vi "arm control.vi"(1 "State":T1, 2 "Z Axis (Tuning)":dbl) -> (0 "setpoint":dbl format="%.2f")   [LabVIEW 2013]
uses:
  typedefs/subStates.ctl
  typedefs/fg_typedef.ctl
panel:
  in  "lower limit":dbl=-0.015 format="%#_13g"
  in  "upper limit":dbl=0.015 format="%#_13g"
  in  "2nd Up setpoint":dbl format="%#_13g"
  in  "1st Up setpoint":dbl format="%#_13g"
  # "Things needing Tuning"
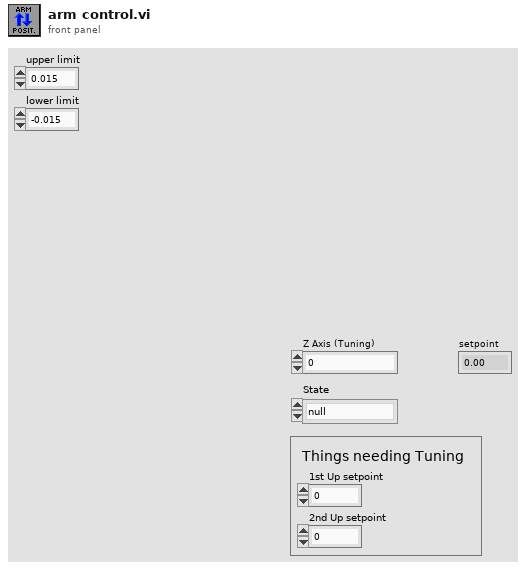
[diagram p1: front panel]
types:
  T1 = typedef "subStates.ctl" = enum16{"null", "wait", "driver control", "auto", "manual override", "hold position", "rotate", "pickup", "pass", "load", "goto shoot", "shoot", "end"}
  T2 = typedef "fg_typedef.ctl" = enum16{"Get", "Set"}
  T3 = typedef "WPI_DigitalInputDevRef.ctl" = cluster{"DevStatus":errorcluster, "DIO Channel":T4, "Digital Module":T5}
  T4 = typedef "FPGA_DIOChannel.ctl" = enum8{"DIO 1", "DIO 2", "DIO 3", "DIO 4", "DIO 5", "DIO 6", "DIO 7", "DIO 8", "DIO 9", "DIO 10", "DIO 11", "DIO 12", "DIO 13", "DIO 14", "Invalid"}
  T5 = typedef "FPGA_TypedefDigitalModule.ctl" = enum16{"Digital Module 1", "Digital Module 2"}
  T6 = typedef "WPI_EncoderDevRef.ctl" = cluster{"DevStatus":errorcluster, "EncoderIndex":T7, "CounterIndex":T8, "DistancePerCount":dbl, "Decoding Type":T9}
  T7 = typedef "FPGA_EncoderIdx.ctl" = enum8{"Enc 0", "Enc 1", "Enc 2", "Enc 3", "Invalid"}
  T8 = typedef "FPGA_CounterCtrSystemIndex.ctl" = enum8{"Ctr 0", "Ctr 1", "Ctr 2", "Ctr 3", "Ctr 4", "Ctr 5", "Ctr 6", "Ctr 7", "Invalid"}
  T9 = typedef "WPI_EncoderType.ctl" = enum16{"1x", "2x", "4x"}
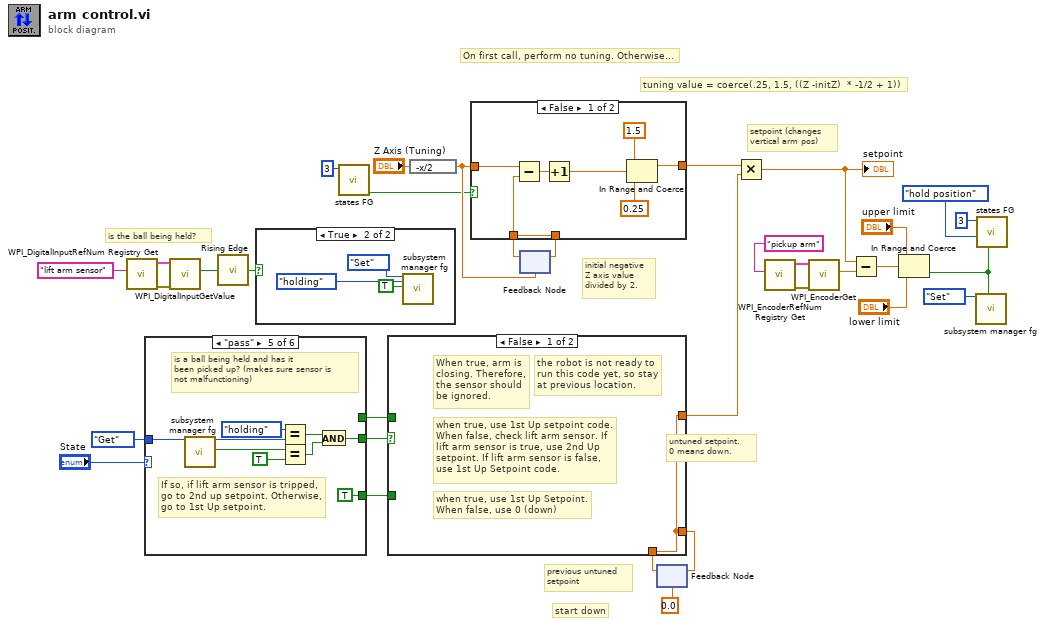
[diagram p0: block diagram]
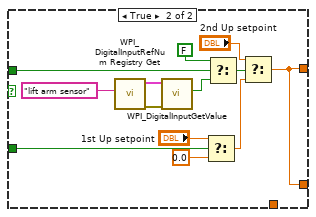
[diagram p3: hidden frame]
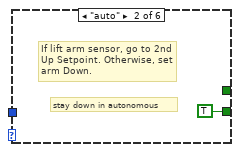
[diagram p5: hidden frame]
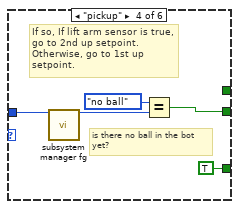
[diagram p7: hidden frame]
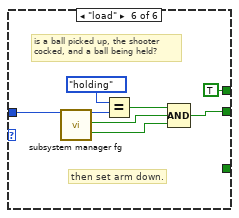
[diagram p8: hidden frame]
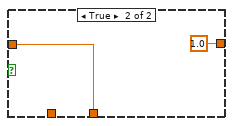
[diagram p9: hidden frame]
diagram:
  # "untuned setpoint.\n0 means down."
  # "tuning value = coerce(.25, 1.5, ((Z -initZ)  * -1/2 + 1))"
  # "initial negative\nZ axis value\ndivided by 2."
  # "On first call, perform no tuning. Otherwise..."
  # "is the ball being held?"
  # "start down"
  # "previous untuned\nsetpoint"
  # "setpoint (changes\nvertical arm pos)"
  n1 = call <vilib>:"WPI_DigitalInputRefNum Registry Get.vi"("refnum name"="lift arm sensor") -> ("error out"=w1:errorcluster, "DigitalInputDevRef"=w2:T3)  [unwired: 9 in]
  n2 = case shown="\"pass\"" "State" {
    tunnel: fg_typedef."Get" ("Menu") -> [_ _ _ w39 w48 w56]
    tunnel: [_ TRUE _ w38 w43 w55] -> w18
    tunnel: [_ _ _ TRUE ("y") TRUE ("y") _] -> w16
    tunnel: [_ _ _ _ _ TRUE ("y")] -> w6
    frame "driver control", Default {
      # "code does not run"
    }
    frame "auto" {
      # "If lift arm sensor, go to 2nd\nUp Setpoint. Otherwise, set\narm Down."
      # "stay down in autonomous"
    }
    frame "manual override" {
      # "code does not run"
    }
    frame "pickup" {
      # "If so, If lift arm sensor is true,\ngo to 2nd up setpoint.\nOtherwise, go to 1st up\nsetpoint."
      # "is there no ball in the bot\nyet?"
      n3 = call "subsystem manager fg.vi"("Menu"=w39) -> ("Ball State Read"=w36:enum16{"no ball", "holding", "loaded"})  [unwired: 14 in, 4 out]
      n4 = Equal?(x=enum16{"no ball", "holding", "loaded"}."no ball" ("y"), y=w36) -> (x = y?=w38:bool)
    }
    frame "pass" {
      # "If so, if lift arm sensor is tripped,\ngo to 2nd up setpoint. Otherwise,\ngo to 1st Up setpoint."
      # "is a ball being held and has it\nbeen picked up? (makes sure sensor is\nnot malfunctioning)"
      n5 = call "subsystem manager fg.vi"("Menu"=w48) -> ("Ball State Read"=w41:enum16{"no ball", "holding", "loaded"}, "Picked Up"=w47:bool)  [unwired: 14 in, 3 out]
      n6 = Equal?(x=enum16{"no ball", "holding", "loaded"}."holding" ("y"), y=w41) -> (x = y?=w44:bool)
      n7 = Equal?(x=w47, y=TRUE) -> (x = y?=w45:bool)
      n8 = And(x=w44, y=w45) -> (x .and. y?=w43:bool)
    }
    frame "load" {
      # "then set arm down."
      # "is a ball picked up, the shooter\ncocked, and a ball being held?"
      n9 = call "subsystem manager fg.vi"("Menu"=w56) -> ("Ball State Read"=w54:enum16{"no ball", "holding", "loaded"}, "Picked Up"=w50:bool, "Shooter Cocked"=w49:bool)  [unwired: 14 in, 2 out]
      n10 = Equal?(x=enum16{"no ball", "holding", "loaded"}."holding", y=w54) -> (x = y?=w52:bool)
      n11 = Compound Arithmetic op=AND(w52, w50, w49) -> (w55:bool)
    }
  }
  n12 = call <vilib>:"WPI_DigitalInputGetValue.vi"("error in (no error)"=w1, "DigitalInputDevRef"=w2) -> ("Value"=w4:bool)  [unwired: 7 in, 2 out]
  n13 = call "Rising Edge.vi"("Input"=w4) -> ("Rising Edge"=w5:bool)
  n14 = case shown="True" w5 {
    frame False {
    }
    frame True {
      n15 = call "subsystem manager fg.vi"("Menu"=fg_typedef."Set", "Ball State Write"=enum16{"no ball", "holding", "loaded"}."holding", "Picked Up"=TRUE) -> ()  [unwired: 12 in, 5 out]
    }
  }
  n16 = call "states FG.vi"("Loop ID"=3) -> ("first call?"=w22:bool)  [unwired: 7 in, 3 out]
  n17 = expression code="-x/2"("Z Axis (Tuning)") -> (w33:dbl)
  n18 = feedback #1(w33) -> (w31:dbl)
  n19 = case shown="False" w22 {
    tunnel: w33 -> [w66 w68]
    tunnel: [w61 w68] -> w30
    tunnel: w31 -> [w61 _]
    tunnel: [w63 1.0 ("upper limit")] -> w17
    frame False {
      n20 = Subtract(x=w66, y=w61) -> (x-y=w62:dbl)
      n21 = Increment(x=w62) -> (x+1=w60:dbl)
      n22 = In Range and Coerce(upper limit=1.5, x=w60, lower limit=0.25) -> (coerced(x)=w63:dbl)  [unwired: 1 out]
    }
    frame True {
    }
  }
  n23 = feedback-in #1(w30) -> ()
  n24 = feedback #2(0.0 ("x")) -> (w8:dbl)
  n25 = case shown="False" w18 {
    tunnel: w16 -> [_ w80]
    tunnel: [w69 w70] -> w10
    tunnel: [w69 w70] -> w9
    tunnel: w8 -> [w69 _]
    tunnel: w6 -> [_ w76]
    frame False {
      # "when true, use 1st Up Setpoint.\nWhen false, use 0 (down)"
      # "when true, use 1st Up setpoint code.\nWhen false, check lift arm sensor. If\nlift arm sensor is true, use 2nd Up\nsetpoint. If lift arm sensor is false,\nuse 1st Up Setpoint code."
      # "When true, arm is\nclosing. Therefore,\nthe sensor should\nbe ignored."
      # "the robot is not ready to\nrun this code yet, so stay\nat previous location."
    }
    frame True {
      n26 = call <vilib>:"WPI_DigitalInputRefNum Registry Get.vi"("refnum name"="lift arm sensor") -> ("error out"=w77:errorcluster, "DigitalInputDevRef"=w78:T3)  [unwired: 9 in]
      n27 = call <vilib>:"WPI_DigitalInputGetValue.vi"("error in (no error)"=w77, "DigitalInputDevRef"=w78) -> ("Value"=w75:bool)  [unwired: 7 in, 2 out]
      n28 = Select(t="1st Up setpoint", s=w80, f=0.0 ("x")) -> (s? t:f=w71:dbl)
      n29 = Select(t=FALSE, s=w76, f=w75) -> (s? t:f=w73:bool)
      n30 = Select(t="2nd Up setpoint", s=w73, f=w71) -> (s? t:f=w70:dbl)
    }
  }
  n31 = feedback-in #2(w9) -> ()
  n32 = Multiply(x=w17, y=w10) -> (x*y=w15:dbl)
  "setpoint" <- w15
  n33 = call <vilib>:"WPI_EncoderRefNum Registry Get.vi"("refnum name"="pickup arm") -> ("error out"=w23:errorcluster, "EncoderDevRef"=w24:T6)  [unwired: 9 in]
  n34 = call <vilib>:"WPI_EncoderGet.vi"("error in (no error)"=w23, "EncoderDevRef"=w24) -> ("Distance"=w29:dbl)  [unwired: 4 in, 5 out]
  n35 = Subtract(x=w15, y=w29) -> (x-y=w26:dbl)
  n36 = In Range and Coerce(upper limit="upper limit", x=w26, lower limit="lower limit") -> (In Range?=w12:bool)  [unwired: 1 out]
  n37 = call "subsystem manager fg.vi"("Menu"=fg_typedef."Set", "Arm Ready"=w12) -> ()  [unwired: 13 in, 5 out]
  n38 = call "states FG.vi"("exit in"=w12, "subState in"=subStates."hold position", "Loop ID"=3) -> ()  [unwired: 5 in, 4 out]
